vi "GetLed.vi"(0 "reference in":refnum<class "LedState.lvclass">, 5 "error in (no error)":errorcluster) -> (14 "reference out":refnum<class "LedState.lvclass">, 16 "Led":bool, 19 "error out":errorcluster)   [LabVIEW 2014, in "LedState.lvclass"]
uses:
  LedState.lvclass
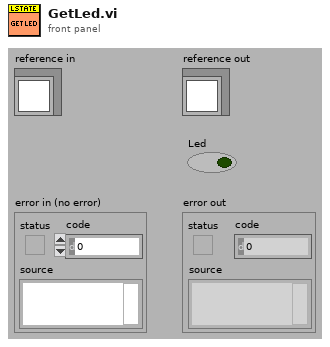
[diagram p1: front panel]
types:
  T1 = typedef "LedState.lvclass/ObjectAttributes.ctl" = cluster{"Led":bool}
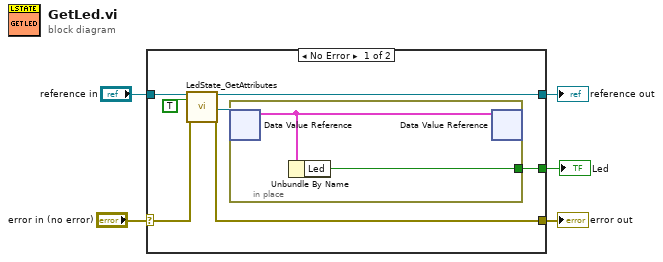
[diagram p0: block diagram]
diagram:
  n1 = case shown="No Error" "error in (no error)" {
    selector: "error in (no error)" -> [w12 w16]
    tunnel: [w11 w16] -> w4
    tunnel: [w9 w15] -> w2
    tunnel: "reference in" -> [w10 w15]
    tunnel: [w6 _] -> w1
    frame No Error {
      n2 = call "LedState_GetAttributes.vi"("reference in"=w10, "OnlyGetDvrReference(False)"=TRUE, "error in (no error)"=w12) -> ("reference out"=w9:refnum<class "LedState.lvclass">, "DataRef"=w8:refnum<data-value>, "error out"=w11:errorcluster)  [unwired: 13 in, 1 out]
      n3 = in-place {
        in-place-border: [w14] -> w6
        n4 = in-place-dvr #1(w8) -> (w13:T1)  [unwired: 1 out]
        n5 = Unbundle By Name(w13) -> ("Led"=w14:bool)
        n6 = in-place-dvr #1(w13) -> ()  [unwired: 2 out]
      }
    }
    frame Error {
    }
  }
  "error out" <- w4
  "reference out" <- w2
  "Led" <- w1
